vi "X-Ray Tube.vi"(8 "error in (no error)":errorcluster) -> (0 "error out":errorcluster, 3 "SceneObject out":refnum<vi>)   [LabVIEW 2026, in "XRay CArm.lvclass"]
uses:
  XRay CArm.lvclass
  <vilib>/picture/3D Picture Control/Object/Create Object (drawable).vi
  <vilib>/picture/3D Picture Control/Object/Add Object (reference).vi
  <vilib>/picture/3D Picture Control/NI_3D Picture Control.lvlib
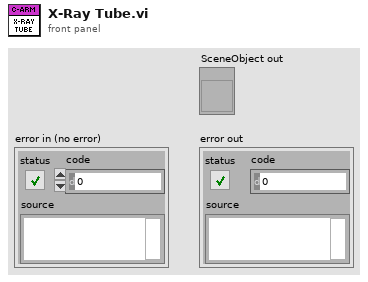
[diagram p1: front panel]
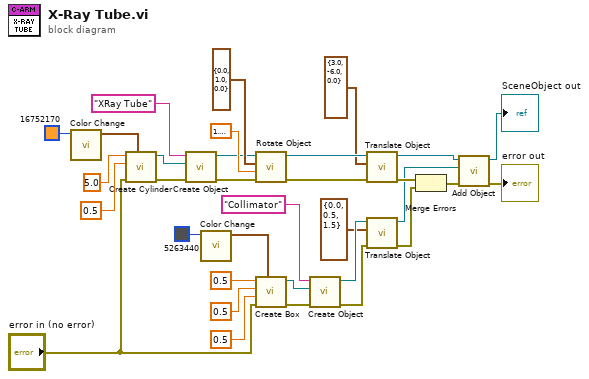
[diagram p0: block diagram]
diagram:
  n1 = call <vilib>:"Color Change.vi"("Color"=u32 16752170) -> ("RGBA"=w2:cluster{"R":sgl, "G":sgl, "B":sgl, "A":sgl})  [unwired: 10 in]
  n2 = call <vilib>:"Create Cylinder.vi"("Color"=w2, "error in (no error)"="error in (no error)", "Radius"=sgl 0.5, "Height"=sgl 5.0) -> ("error out"=w8:errorcluster, "New Cylinder Refnum"=w7:refnum<vi>)  [unwired: 6 in]
  n3 = call-poly <vilib>:"Create Object.vi"("error in (no error)"=w8, "Geometry"=w7, "Name"="XRay Tube") -> ("error out"=w25:errorcluster, "Scene:New Object"=w9:refnum<vi>)  [unwired: 7 in]
  n4 = call <vilib>:"Color Change.vi"("Color"=u32 5263440) -> ("RGBA"=w21:cluster{"R":sgl, "G":sgl, "B":sgl, "A":sgl})  [unwired: 10 in]
  n5 = call <vilib>:"Rotate Object.vi"("error in (no error)"=w25, "Angle"=1.5707963267948966, "Axis"=cluster{"X":sgl, "Y":sgl, "Z":sgl} {"X"=0.0, "Y"=1.0, "Z"=0.0}, "Scene.Object In"=w9) -> ("error out"=w26:errorcluster, "Scene.Object Out"=w10:refnum<vi>)  [unwired: 6 in]
  n6 = call <vilib>:"Create Box.vi"("Color"=w21, "error in (no error)"="error in (no error)", "Length Z"=sgl 0.5 ("Box Length Z"), "Length Y"=sgl 0.5 ("Box Length Y"), "Length X"=sgl 0.5 ("Box Length X")) -> ("error out"=w20:errorcluster, "New Box Refnum"=w19:refnum<vi>)  [unwired: 5 in]
  n7 = call-poly <vilib>:"Create Object.vi"("error in (no error)"=w20, "Geometry"=w19, "Name"="Collimator") -> ("error out"=w28:errorcluster, "Scene:New Object"=w18:refnum<vi>)  [unwired: 7 in]
  n8 = call <vilib>:"Translate Object.vi"("error in (no error)"=w26, "Translation"=cluster{"X":sgl, "Y":sgl, "Z":sgl} {"X"=3.0, "Y"=-6.0, "Z"=0.0} ("Translation 4"), "Scene.Object In"=w10) -> ("error out"=w30:errorcluster, "Scene.Object Out"=w24:refnum<vi>)  [unwired: 7 in]
  n9 = call <vilib>:"Translate Object.vi"("error in (no error)"=w28, "Translation"=cluster{"X":sgl, "Y":sgl, "Z":sgl} {"X"=0.0, "Y"=0.5, "Z"=1.5} ("Translation 3"), "Scene.Object In"=w18) -> ("error out"=w31:errorcluster, "Scene.Object Out"=w27:refnum<vi>)  [unwired: 7 in]
  n10 = Merge Errors(w30, w31) -> (w32:errorcluster)
  n11 = call-poly <vilib>:"Add Object.vi"("error in (no error)"=w32, "New Object In"=w27, "Scene Object In"=w24) -> ("error out"=→"error out":errorcluster, "Scene Object Out"=→"SceneObject out":refnum<vi>)  [unwired: 6 in, 1 out]
